vi "Read Word Log Producer.vi"(8 "error in (no error)":errorcluster, 11 "Shared Resources in":refnum<class "Shared Resources.lvclass">) -> (0 "error out":errorcluster, 2 "Communication Bus Template Interfaces:Implementation.lvlib:Logging.lvlib:Word Log Producer.lvclass":refnum<class "Word Log Producer.lvclass">, 3 "Shared Resources out":refnum<class "Shared Resources.lvclass">)   [LabVIEW 2020, in "Ballard ARINC 429 Engine.lvlib" / "Implementation.lvlib" / "Shared Resources.lvclass"]
uses:
  Shared Resources.lvclass
  Logging/Word Log Producer/Word Log Producer.lvclass
  Shared Resources.lvclass/Shared Resources.ctl
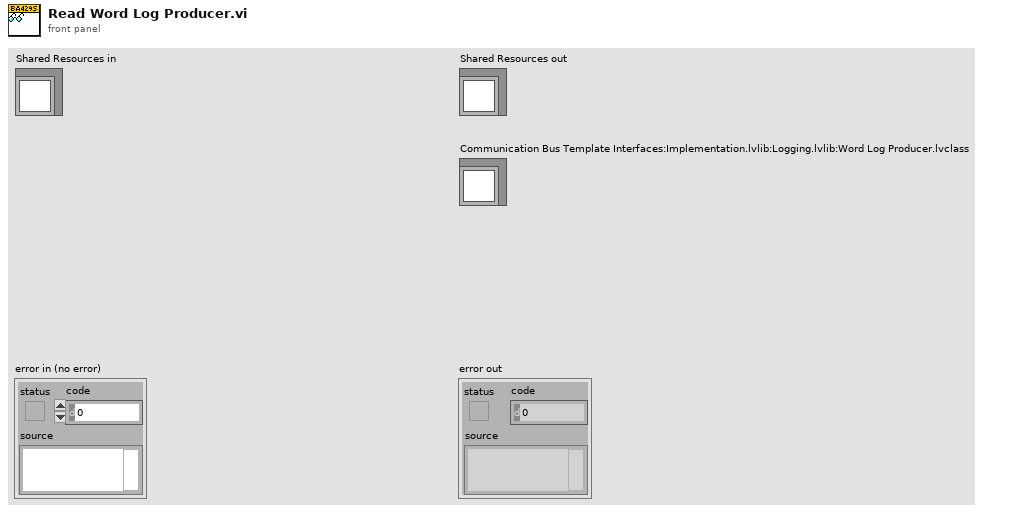
[diagram p1: front panel]
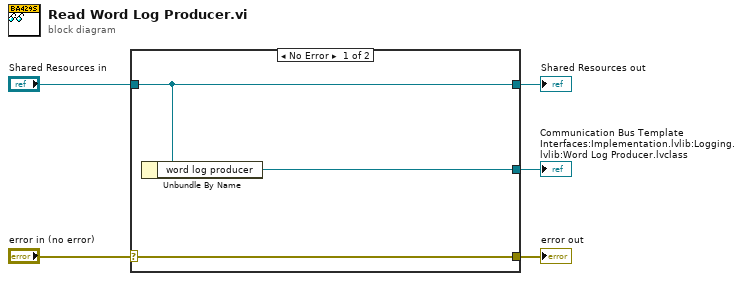
[diagram p0: block diagram]
diagram:
  n1 = case shown="No Error" "error in (no error)" {
    selector: "error in (no error)" -> [w8 w9]
    tunnel: [w8 w9] -> w4
    tunnel: [w7 w10] -> w2
    tunnel: "Shared Resources in" -> [w7 w10]
    tunnel: [w6 _] -> w1
    frame No Error {
      n2 = Unbundle By Name(w7) -> ("word log producer"=w6:refnum<class "Word Log Producer.lvclass">)
    }
    frame Error {
    }
  }
  "error out" <- w4
  "Shared Resources out" <- w2
  "Communication Bus Template Interfaces:Implementation.lvlib:Logging.lvlib:Word Log Producer.lvclass" <- w1
